vi "Handle Connection Read Error.vi"(7 "Websocket Client Handler in":refnum<class "Websocket Client Handler.lvclass">, 8 "error in (no error)":errorcluster, 11 "Self Enqueuer":refnum<class "Message Transport Queue.lvclass">) -> (0 "error out":errorcluster, 5 "Websocket Client Handler out":refnum<class "Websocket Client Handler.lvclass">)   [LabVIEW 2016, in "Stream Mediator.lvlib" / "Websocket Client Handler.lvclass"]
doc: "--\nCopyright © 2017 Composed SystemsI All rights reserved.\n\nAuthor: Jon McBee <jon.mcbee@composed.io>\n\nThis library is provided \"AS IS\" ,WITHOUT WARRANTIES OR\nCONDITIONS OF ANY KIND, either express or implied.\n\nComposed Systems -- composed.io\n\nStream 0.0.1.1\nJon McBee - Composed Systems\nCopyright (c) 2017, Composed Systems"
uses:
  <userlib>/Composed Systems/Stream/Mediator/Classes/Websocket Client Handler Actor/Websocket Client Handler/Websocket Client Handler.lvclass
  <userlib>/Composed Systems/Stream/Mediator/Classes/Message Transport Queue/Message Transport Queue.lvclass
  C:/Program Files (x86)/National Instruments/LabVIEW 2016/user.lib/Composed Systems/Stream/Mediator/Classes/Message Transport Interface/Message Transport Interface.lvclass
  <userlib>/Composed Systems/Stream/Mediator/Classes/Message Command Stop/Stop Msg.lvclass
  <userlib>/Composed Systems/Stream/Mediator/Classes/Websocket Client Handler Actor/Websocket Client Handler Msgs/Read Msg/Read Msg.lvclass
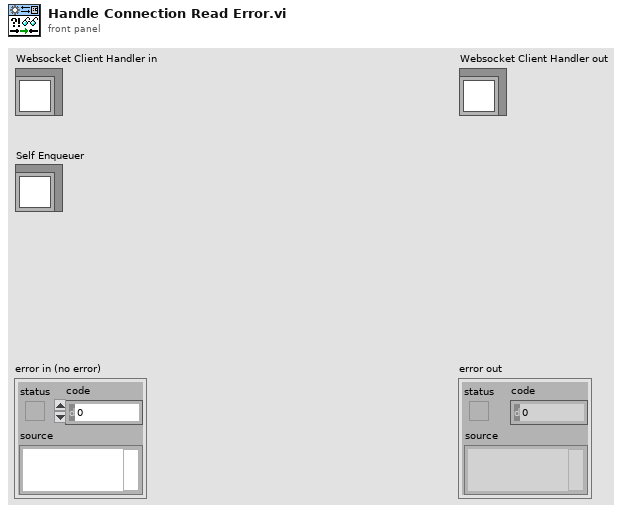
[diagram p1: front panel]
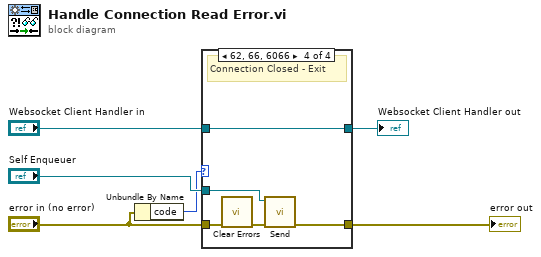
[diagram p0: block diagram]
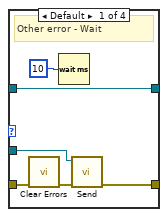
[diagram p2: hidden frame]
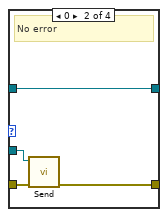
[diagram p3: hidden frame]
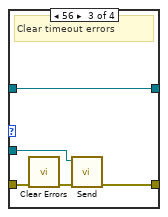
[diagram p4: hidden frame]
diagram:
  n1 = Unbundle By Name("error in (no error)") -> ("code"=w3:i32)
  n2 = case shown="62, 66, 6066" w3 {
    tunnel: [w9 w14 w18 w22] -> w1
    tunnel: "error in (no error)" -> [w10 w15 w21 w26]
    tunnel: [w11 w16 w20 w25] -> w2
    tunnel: "Websocket Client Handler in" -> [w11 w16 w20 w25]
    tunnel: "Self Enqueuer" -> [w8 w13 w17 w24]
    frame Default {
      # "Other error - Wait"
      n3 = call <vilib>:"Clear Errors.vi"("error in (no error)"=w10) -> ("error out"=w7:errorcluster)  [unwired: 5 in, 1 out]
      n4 = Wait (ms)(milliseconds to wait=u32 10) -> ()  [unwired: 1 out]
      n5 = call <userlib>:"Send.vi"("error in (no error)"=w7, "Message Transport Queue"=w8) -> ("error out"=w9:errorcluster)  [unwired: 9 in]
    }
    frame 0 {
      # "No error"
      n6 = call <userlib>:"Send.vi"("error in (no error)"=w15, "Message Transport Queue"=w13) -> ("error out"=w14:errorcluster)  [unwired: 9 in]
    }
    frame 56 {
      # "Clear timeout errors"
      n7 = call <vilib>:"Clear Errors.vi"("error in (no error)"=w21) -> ("error out"=w19:errorcluster)  [unwired: 5 in, 1 out]
      n8 = call <userlib>:"Send.vi"("error in (no error)"=w19, "Message Transport Queue"=w17) -> ("error out"=w18:errorcluster)  [unwired: 9 in]
    }
    frame 62, 66, 6066 {
      # "Connection Closed - Exit"
      n9 = call <vilib>:"Clear Errors.vi"("error in (no error)"=w26) -> ("error out"=w23:errorcluster)  [unwired: 5 in, 1 out]
      n10 = call <userlib>:"Send.vi"("error in (no error)"=w23, "Message Transport"=w24) -> ("error out"=w22:errorcluster)  [unwired: 9 in]
    }
  }
  "error out" <- w1
  "Websocket Client Handler out" <- w2
